vi "check_everything.vi"(0 "VISA引用句柄输入":refnum<visa-resource-name>, 7 "错误输入（无错误）":errorcluster, 8 "数值输入":i32) -> (10 "电压设置回读":string, 12 "数值输出":i32, 14 "电流值回读":string, 16 "蜂鸣器":string, 17 "On/Off":string, 18 "CC/CV":string, 19 "电压值回读":string, 20 "VISA引用句柄输出":refnum<visa-resource-name>, 21 "过压":string, 22 "测量模式":string, 23 "键盘锁":string, 24 "过温":string, 25 "过压设置值回读":string, 26 "电流设置回读":string, 27 "错误输出":errorcluster)   [LabVIEW 2014]
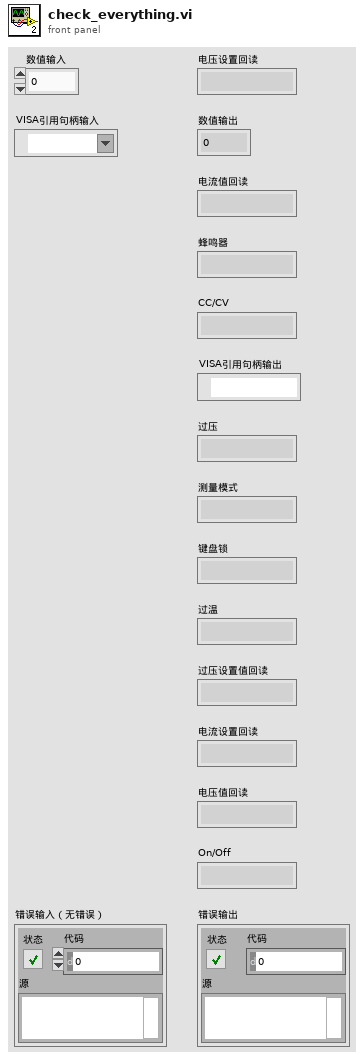
[diagram p1: front panel]
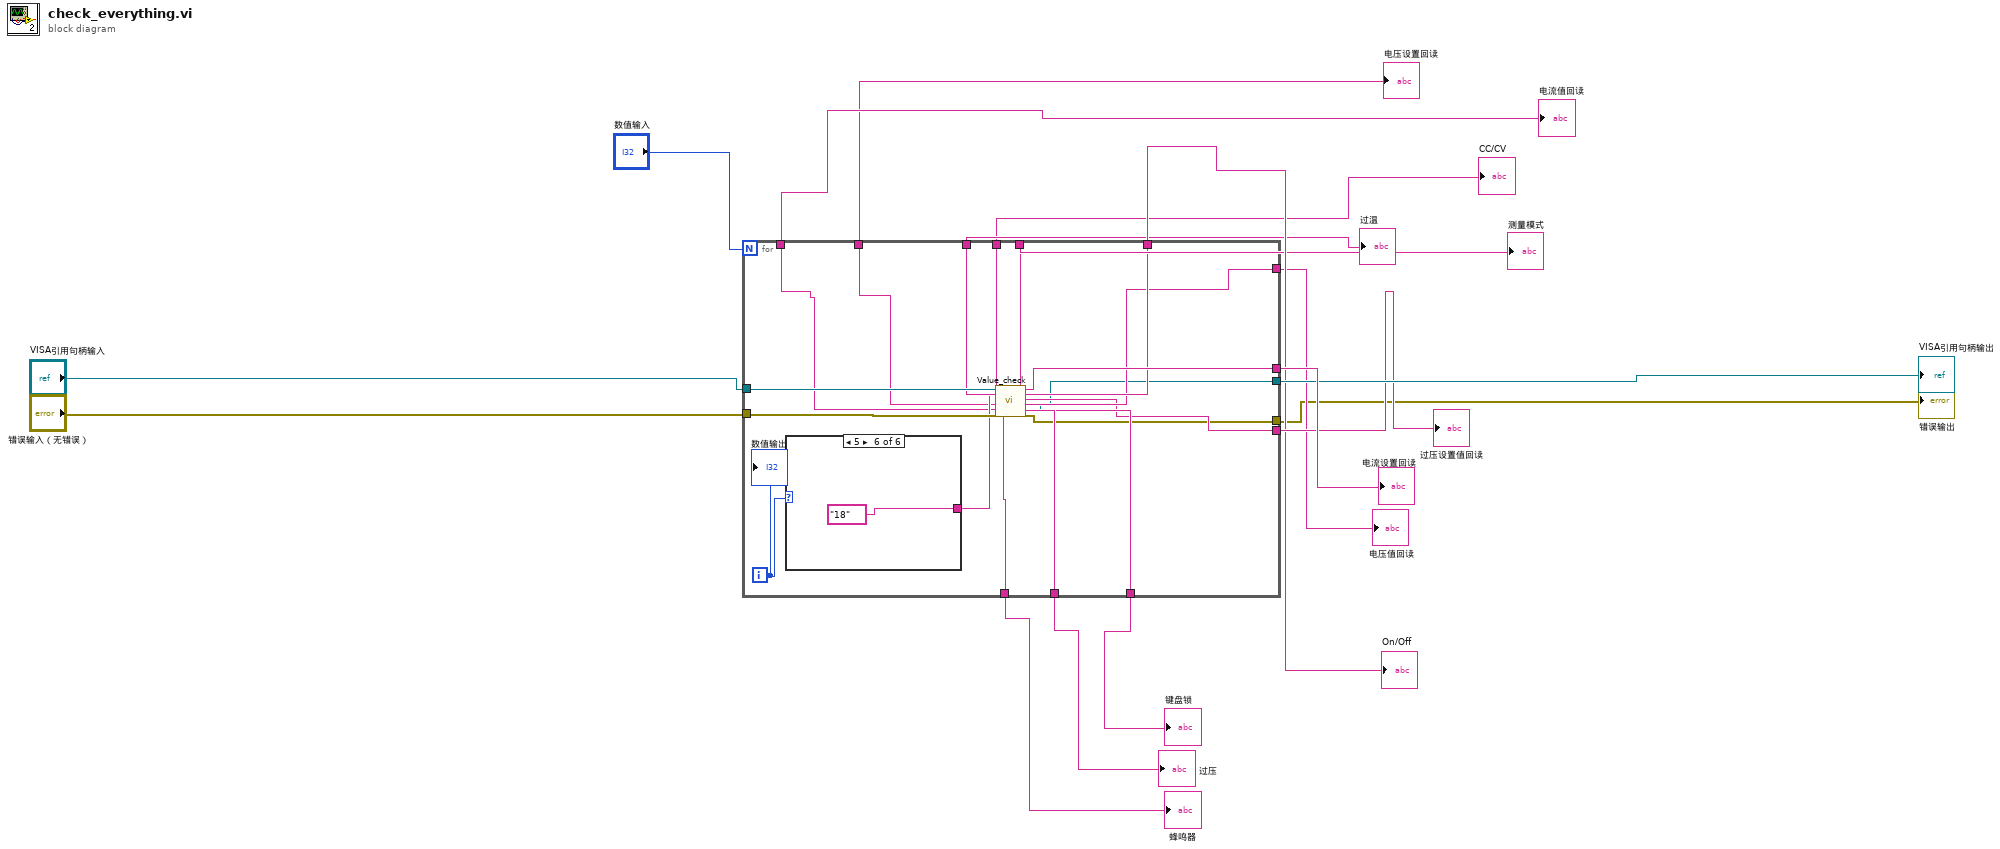
[diagram p0: block diagram]
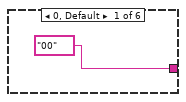
[diagram p2: hidden frame]
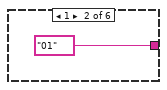
[diagram p3: hidden frame]
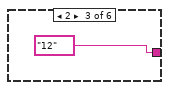
[diagram p4: hidden frame]
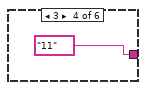
[diagram p5: hidden frame]
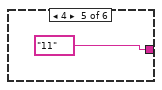
[diagram p6: hidden frame]
diagram:
  n1 = for {
    N: "数值输入" -> [_]
    tunnel: "VISA引用句柄输入" -> [w35]
    tunnel: "错误输入（无错误）" -> [w34]
    tunnel: [w33] -> w15
    tunnel: [w32] -> w9
    tunnel: [w31] -> w7
    tunnel: [w30] -> w6
    tunnel: [w29] -> w5
    tunnel: [w28] -> w12
    tunnel: [w27] -> w11
    tunnel: [w26] -> w10
    tunnel: [w23] -> w4
    tunnel: [w22] -> w3
    tunnel: [w21] -> w8
    tunnel: [w20] -> w13
    tunnel: [w19] -> w2
    tunnel: [w18] -> w14
    i -> [w24]
    n2 = case shown="5" w24 {
      tunnel: ["00" "01" "12" "11" "11" "18"] -> w25
      frame 0, Default {
      }
      frame 1 {
      }
      frame 2 {
      }
      frame 3 {
      }
      frame 4 {
      }
      frame 5 {
      }
    }
    n3 = call "Value_check.vi"("VISA引用句柄输入"=w35, "Status Code"=w25, "错误输入（无错误）"=w34) -> ("电压设置回读"=w22:string, "电流值回读"=w23:string, "过温"=w31:string, "蜂鸣器"=w28:string, "测量模式"=w30:string, "过压"=w27:string, "CC/CV"=w29:string, "键盘锁"=w26:string, "电流设置回读"=w33:string, "On/Off"=w32:string, "过压设置值回读"=w20:string, "电压值回读"=w21:string, "VISA资源名称输出"=w18:refnum<visa-resource-name>, "错误输出"=w19:errorcluster)  [unwired: 3 in]
    "数值输出" <- w24
  }
  "电流设置回读" <- w15
  "VISA引用句柄输出" <- w14
  "过压设置值回读" <- w13
  "蜂鸣器" <- w12
  "过压" <- w11
  "键盘锁" <- w10
  "On/Off" <- w9
  "电压值回读" <- w8
  "过温" <- w7
  "测量模式" <- w6
  "CC/CV" <- w5
  "电流值回读" <- w4
  "电压设置回读" <- w3
  "错误输出" <- w2
